vi "TCP_Write.vi"(0 "String 1":string, 1 "String 4":string, 2 "String 3":string, 3 "String 2":string, 5 "error in (no error) 2":errorcluster) -> (8 "State":bool, 9 "error out":errorcluster)   [LabVIEW 2022 SP3]
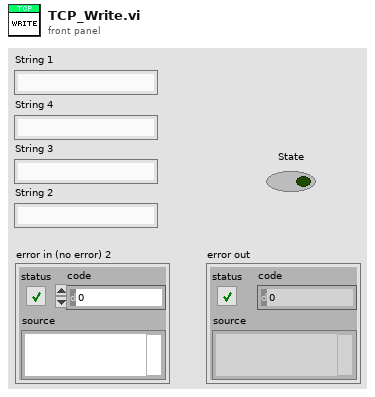
[diagram p1: front panel]
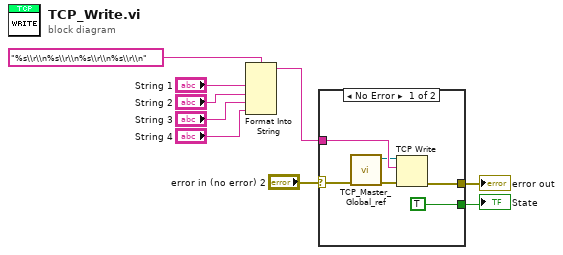
[diagram p0: block diagram]
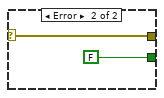
[diagram p2: hidden frame]
diagram:
  n1 = Format Into String(format string="%s\\r\\n%s\\r\\n%s\\r\\n%s\\r\\n", "String 1", "String 2", "String 3", "String 4") -> (resulting string=w4:string)  [unwired: 2 in, 1 out]
  n2 = case shown="No Error" "error in (no error) 2" {
    selector: "error in (no error) 2" -> [w12 w17]
    tunnel: w4 -> [w15 _]
    tunnel: [w11 w17] -> w2
    tunnel: [TRUE ("State") FALSE ("State")] -> w1
    frame No Error {
      n3 = call "TCP_Master_Global_ref.vi"("error in (no error) 2"=w12) -> ("error out 2"=w13:errorcluster, "ID OUT"=w14:refnum<k5>)  [unwired: 9 in]
      n4 = TCP Write(connection ID=w14, data in=w15, error in (no error)=w13) -> (error out=w11:errorcluster)  [unwired: 1 in, 2 out]
    }
    frame Error {
    }
  }
  "error out" <- w2
  "State" <- w1
